vi "transpose string worksheet.vi"() -> ()   [LabVIEW 2024]
panel:
  out "2D or 1D transposed":string
  out "analyzed":string
  in  "field":dbl
  out "1D transposed":string
  in  "?":string
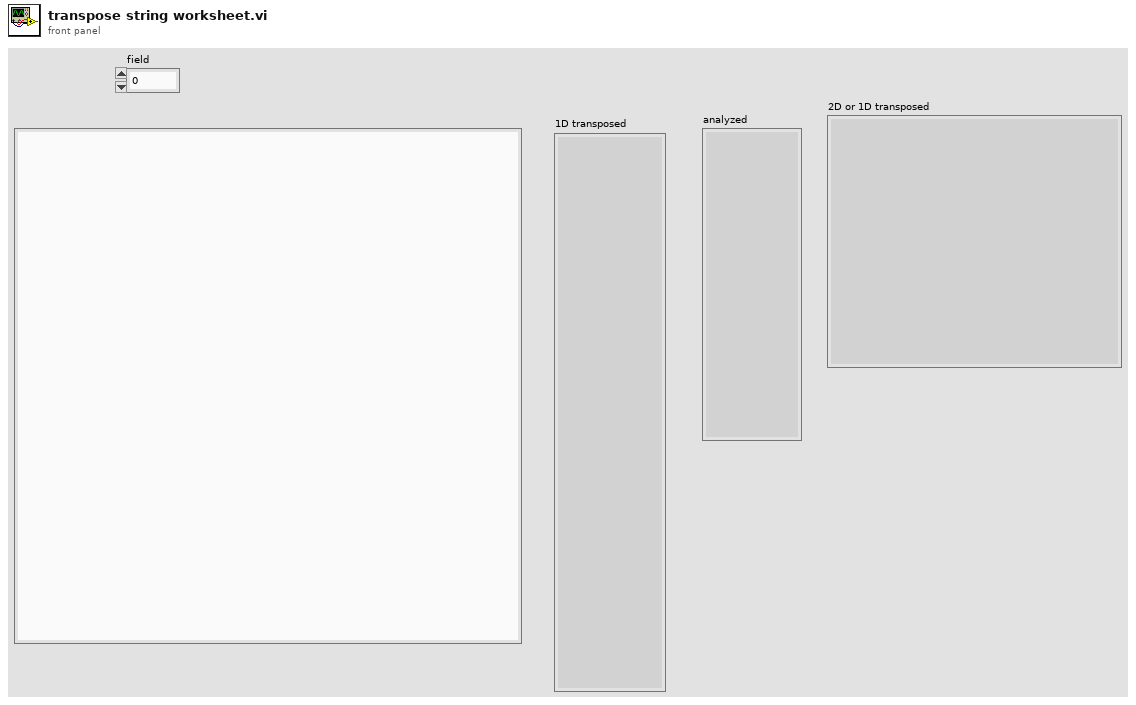
[diagram p1: front panel]
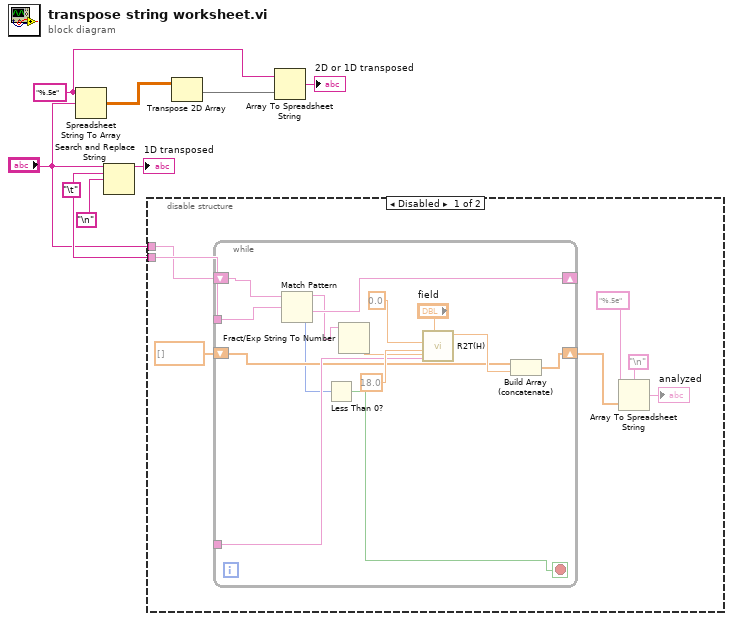
[diagram p0: block diagram]
diagram:
  w2 = "%.5e" ("format string")
  w6 = "\t"
  n1 = Spreadsheet String To Array(format string=w2, spreadsheet string="?") -> (array=w4:dbl[][])  [unwired: 2 in]
  n2 = Search and Replace String(input string="?", search string=w6, replace string="\n") -> (result string=→"1D transposed":string)  [unwired: 5 in, 3 out]
  n3 = disable-structure shown="Disabled" {
    disable-tunnel: w6 -> [w14 _]
    disable-tunnel: "?" -> [w9 _]
    frame Disabled {
      n4 = while {
        shift-right: [w28] -> _
        shift-left: w9 -> [w29]
        tunnel: _ -> [w24]
        shift-right: [w20] -> w13
        shift-left: dbl[] [] -> [w19]
        tunnel: w14 -> [w16]
        stop <- w17 stop-if-true
        n5 = Match Pattern(string=w29, regular expression=w16) -> (before substring=w27:string, after substring=w28:string, offset past match=w18:i32)  [unwired: 1 in, 1 out]
        n6 = Less Than 0?(x=w18) -> (x < 0?=w17:bool)
        n7 = Fract/Exp String To Number(string=w27) -> (number=w22:dbl)  [unwired: 3 in, 1 out]
        n8 = call "R2T(H).vi"("input"=w22, "field"="field", "master coeff"=w24, "end H"=18.0, "start H"=0.0) -> ("output"=w21:dbl)  [unwired: 6 in]
        n9 = Build Array (concatenate)(w19, w21) -> (w20:dbl[])
      }
      n10 = Array To Spreadsheet String(delimiter (Tab)="\n", array=w13, 3:"%.5e" ("format string")) -> (spreadsheet string=→"analyzed":string)
    }
    frame Enabled {
    }
  }
  n11 = Transpose 2D Array(2D array=w4) -> (transposed array=w3:dbl[][])
  n12 = Array To Spreadsheet String(array=w3, 3:w2) -> (spreadsheet string=→"2D or 1D transposed":string)  [unwired: 1 in]
